vi "(SubVI) Monitor DNA length.vi"(5 "OK Button":bool caption="Reset BM", 6 "initial parameters":dbl[](array[numeric])=[15.0, 2.0, 15.0, 2.0, 100.0, 127.0], 7 "Input Image":T1(plugin-control)) -> (2 "Results":dbl[](array[numeric]))   [LabVIEW 2014]
panel:
  in  "BMx array in (nm)":dbl[](array[numeric])
  in  "BMy array in (nm)":dbl[](array[numeric])
  in  "y position array in (nm)":dbl[](array[numeric]) format="%0.2f"
  in  "x position array in (nm)":dbl[](array[numeric]) format="%0.2f"
  out "error out":errorcluster
  in  "error in (no error)":errorcluster
  in  "Tab Control":enum32{"DNA", "Image", "Results"}(tab)
  out "BMy array appended (nm)":dbl[](array[numeric])
  out "y position appended array":dbl[](array[numeric])
  out "updated BMy (nm)":dbl
  out "updated BMx (nm)":dbl
  out "BMx array appended (nm)":dbl[](array[numeric])
  out "x position appended array":dbl[](array[numeric])
  out "xy ratio":dbl
  out "y position (nm)":dbl
  out "x position (nm)":dbl
  out "Parameter Names":string[](array[string])=["Xposition", "Xwidth", "Yposition", "Ywidth", "Amplitude", "Offset"]
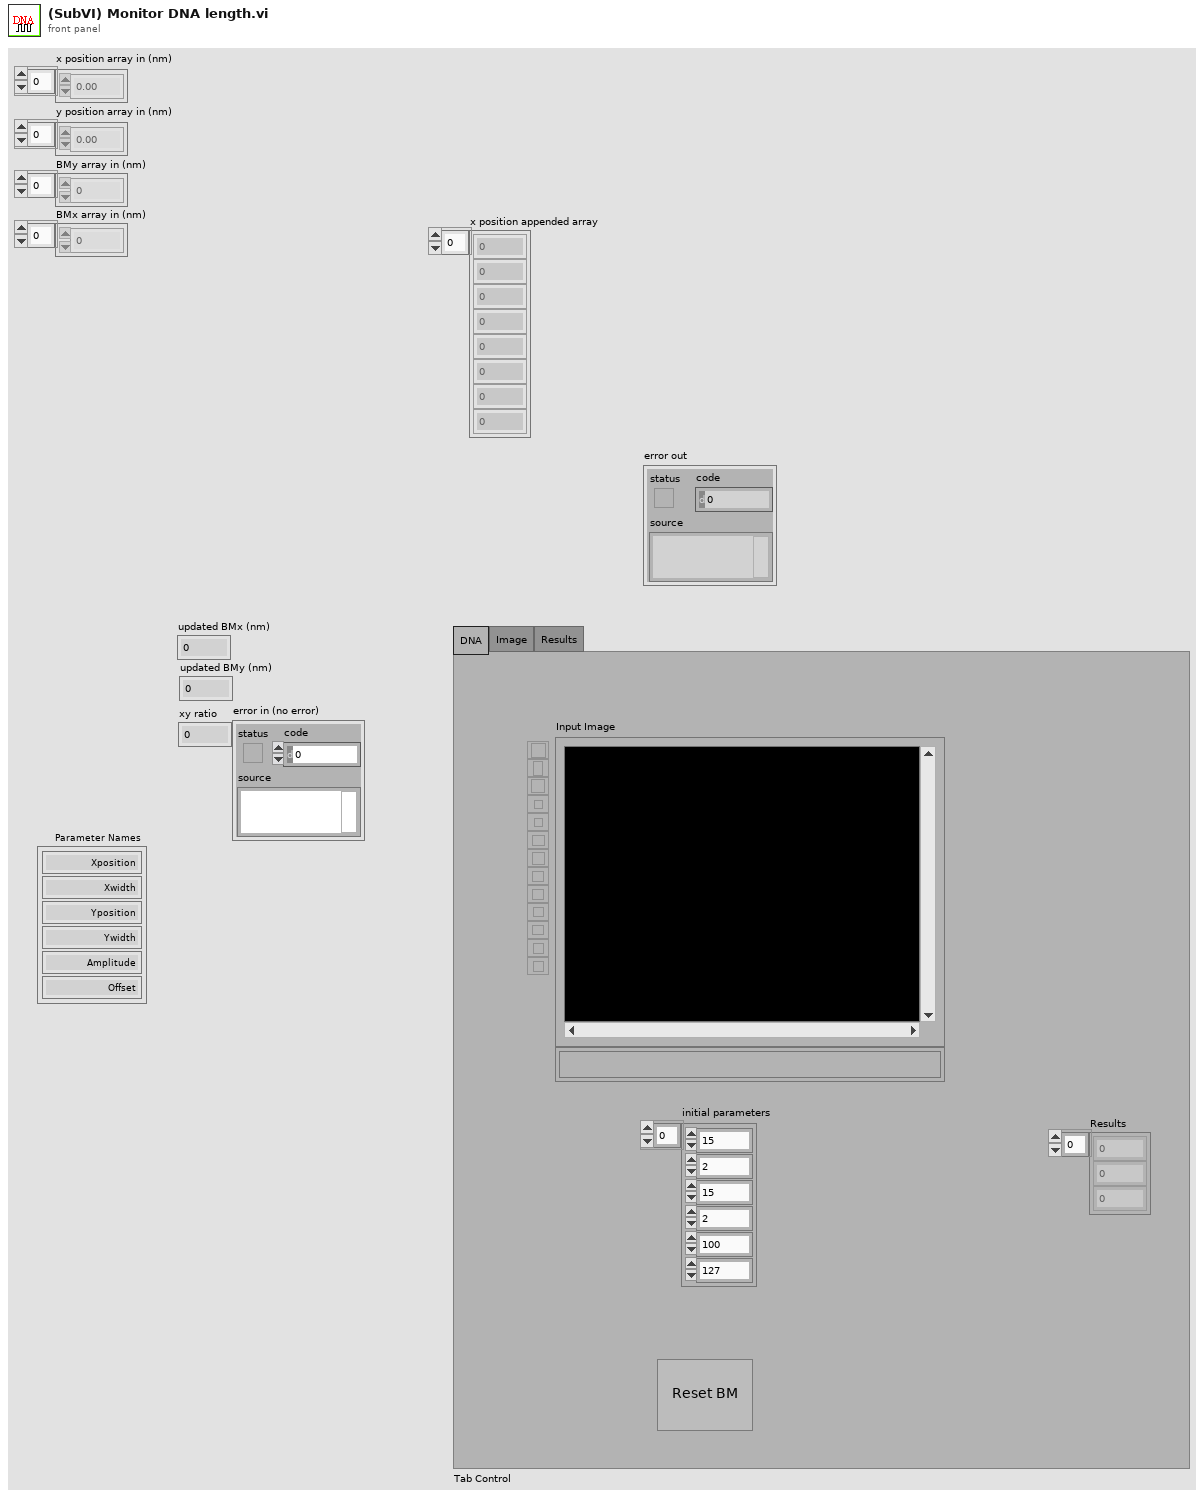
[diagram p1: front panel]
types:
  T1 = typedef "IMAQ Image.ctl" = refnum<image>
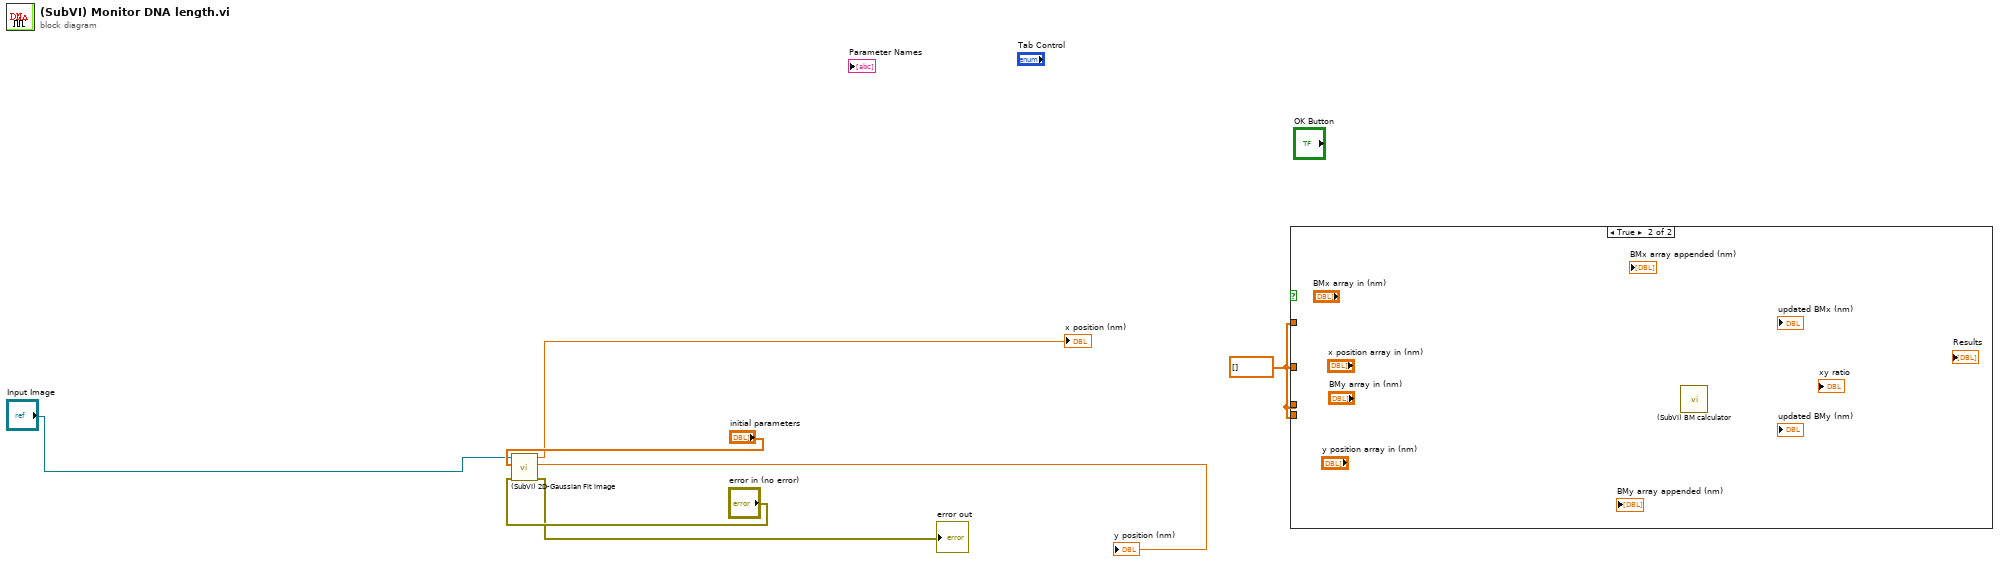
[diagram p0: block diagram]
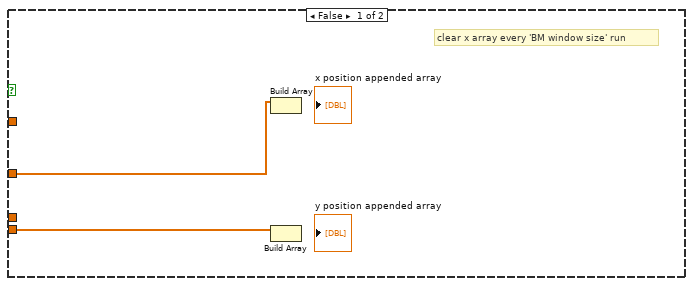
[diagram p2: hidden frame]
diagram:
  w7 = dbl[] []
  n1 = call "(SubVI) 2D-Gaussian Fit image.vi"("error in (no error)"="error in (no error)", "initial parameters"="initial parameters", "Input Image"="Input Image") -> ("error out"=→"error out":errorcluster, "y position (nm)"=→"y position (nm)":dbl, "x position (nm)"=→"x position (nm)":dbl)  [unwired: 6 in]
  n2 = case shown="True" {
    selector: _ -> [_ _]
    tunnel: w7 -> [w9 _]
    tunnel: w7 -> [w8 _]
    tunnel: w7 -> [_ _]
    tunnel: w7 -> [_ _]
    frame False {
      # "clear x array every 'BM window size' run"
      n3 = Build Array(w9) -> ()  [unwired: 1 in, 1 out]
      n4 = Build Array(w8) -> ()  [unwired: 1 in, 1 out]
    }
    frame True {
      n5 = call "(SubVI) BM calculator.vi"() -> ()  [unwired: 12 in]
    }
  }
